vi "Recall Load.vi"(0 "LV MDI in":refnum<class "LV MDI.lvclass">, 9 "LV Serialize[]":refnum<class "MDI serialize.lvclass">[](array[class]), 11 "error in (no error)":errorcluster) -> (4 "LV MDI out":refnum<class "LV MDI.lvclass">, 6 "Doc UID[]":string[](array[string]), 8 "Position[]":T1[](array[typedef]), 10 "Doc UID Displayed[]":string[](array[string]), 15 "error out":errorcluster)   [LabVIEW 2016, in "LV MDI.lvclass"]
doc: "Reload Document Name,Window position and Display status of child windows from XML file."
uses:
  LV MDI.lvclass
  protected/Postion.ctl
  MDI serialize/MDI serialize.lvclass
  LV MDI.lvclass/LV MDI.ctl
  Document/Document base/Document.lvclass/Document.ctl
  MDI serialize/MDI serialize.lvclass/MDI serialize.ctl
  Document/Document base/property/Read Doc UID.vi
  Document/Document base/property/Read Doc Title.vi
  MDI serialize/property/Read Document Name.vi
  MDI serialize/property/Read Show Window.vi
  MDI serialize/property/Read Child Position.vi
  Document/Document base/Document.lvclass
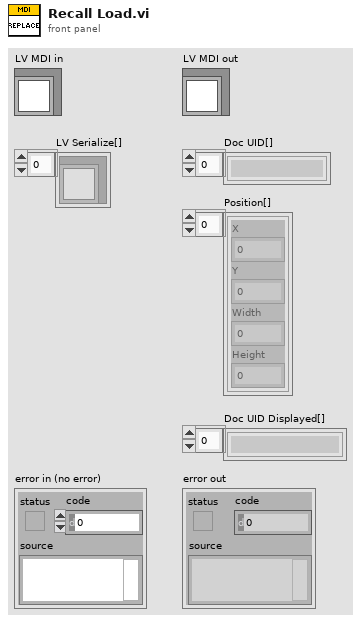
[diagram p1: front panel]
types:
  T1 = typedef "Postion.ctl" = cluster{"X":i32, "Y":i32, "Width":i32, "Height":i32}
  T2 = typedef "LV MDI.lvclass/Postion.ctl" = cluster{"X":i32, "Y":i32, "Width":i32, "Height":i32}
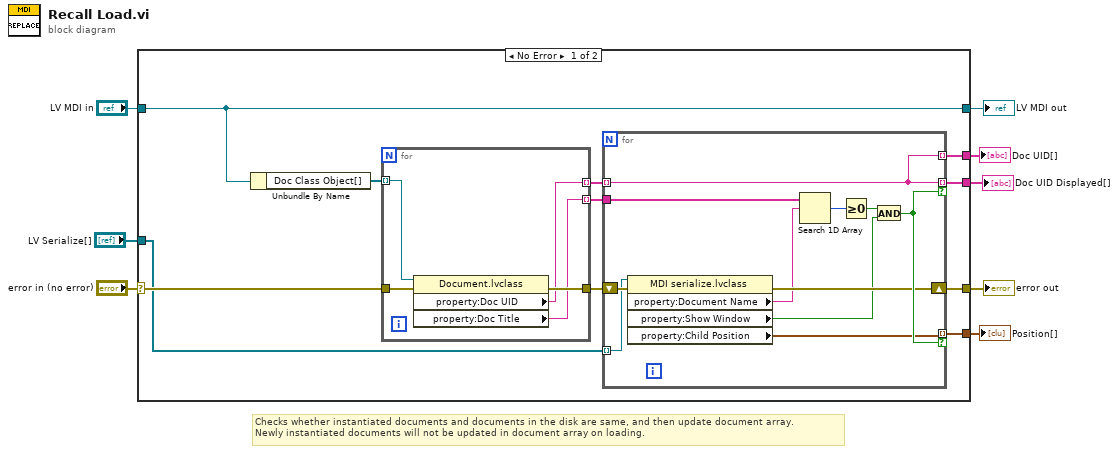
[diagram p0: block diagram]
diagram:
  # "Checks whether instantiated documents and documents in the disk are same, and then update document array.\nNewly instantiated documents will not be updated in document array on loading."
  n1 = case shown="No Error" "error in (no error)" {
    selector: "error in (no error)" -> [w19 w37]
    tunnel: [w15 w37] -> w7
    tunnel: [w17 w36] -> w5
    tunnel: "LV MDI in" -> [w17 w36]
    tunnel: "LV Serialize[]" -> [w10 _]
    tunnel: [w12 _] -> w4
    tunnel: [w11 _] -> w3
    tunnel: [w9 _] -> w1
    frame No Error {
      n2 = Unbundle By Name(w17) -> ("Doc Class Object[]"=w18:refnum<class "Document.lvclass">[])
      n3 = for {
        tunnel: w19 -> [w35]
        tunnel: [w34] -> w16
        tunnel: w18 -> [w33] mode=indexing
        tunnel: [w32] -> w14 mode=indexing
        tunnel: [w31] -> w13 mode=indexing
        n4 = property class="Document.lvclass"(reference=w33, error in=w35) -> (error out=w34:errorcluster, "property:Doc UID"=w31:string, "property:Doc Title"=w32:string)  [unwired: 1 out]
      }
      n5 = for {
        tunnel: w14 -> [w28]
        shift-right: [w24] -> w15
        shift-left: w16 -> [w30]
        tunnel: w13 -> [w25] mode=indexing
        tunnel: [w25] -> w12 mode=indexing if=w26
        tunnel: [w20] -> w9 mode=indexing if=w26
        tunnel: [w25] -> w11 mode=indexing
        tunnel: w10 -> [w23] mode=indexing
        n6 = property class="MDI serialize.lvclass"(reference=w23, error in=w30) -> (error out=w24:errorcluster, "property:Document Name"=w22:string, "property:Show Window"=w21:bool, "property:Child Position"=w20:T2)  [unwired: 1 out]
        n7 = Search 1D Array(1D array=w28, element=w22) -> (index of element=w29:i32)  [unwired: 1 in]
        n8 = Greater Or Equal To 0?(x=w29) -> (x >= 0?=w27:bool)
        n9 = And(x=w27, y=w21) -> (x .and. y?=w26:bool)
      }
    }
    frame Error {
    }
  }
  "error out" <- w7
  "LV MDI out" <- w5
  "Doc UID Displayed[]" <- w4
  "Position[]" <- w1
  "Doc UID[]" <- w3
